vi "temperature.vi"(8 "Numérique":dbl) -> (0 "Thermomètre":dbl(slide) scale=-20.0..50.0)   [LabVIEW 2017]
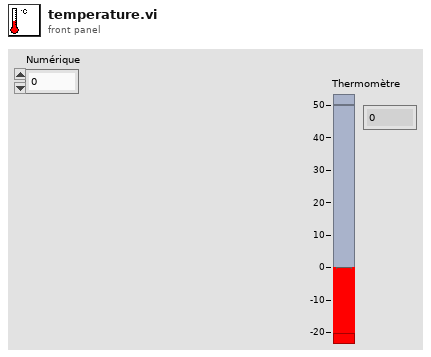
[diagram p1: front panel]
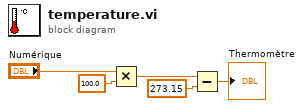
[diagram p0: block diagram]
diagram:
  n1 = Multiply(x="Numérique", y=100.0) -> (x*y=w3:dbl)
  n2 = Subtract(x=w3, y=273.15) -> (x-y=→"Thermomètre":dbl)
